vi "Official Gyro Example.vi"() -> ()   [LabVIEW 2016]
doc: "This example is for the HiTechnic Gyro Sensor together with the LEGO MINDSTORMS NXT. This program shows the angular rate on the NXT screen as well as on the Front Panel with a gauge indicator."
uses:
  <vilib>/NXT/HiTechnic/HiTechnic Controls/HiTechnic Port.ctl
  <vilib>/NXT/Block Support/NXT_InputPort.ctl
  <vilib>/NXT/Dual Mode Library/Display/drawText.vi
panel:
  out "Offset Value":i16
  in  "Reset Button":bool
  in  "stop":bool
  out "Gauge":i16(knob) scale=-360.0..360.0
  # "HiTechnic Gyro"
  # "Description\n\nThis example shows the HiTechnic Gyro Sensor value on the NXT screen on and this Front Panel gauge.  Pressing the Reset Offset button or the NXT Enter button will reset the Offset based on the current sensor reading.\n\nPorts\nPort 1: HiTechnic Gyro Sensor\n\n\nFor additional information: www.hitechnic.com"
  # "Controls and Indicators\n\nGauge shows the current Gyro Sensor value.  The units are in degrees/second.\n\nIf the sensor value is non-zero even when the sensor is not turning, press the Reset Offset button to adjust the offset."
  # "deg/sec"
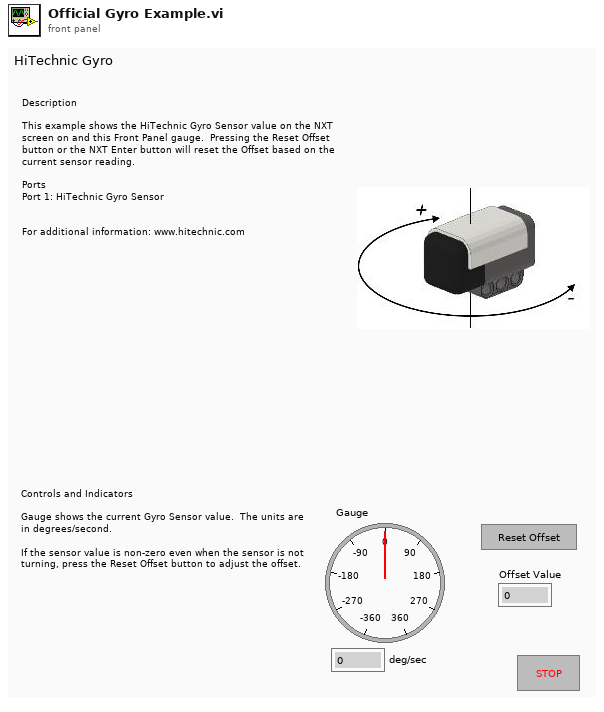
[diagram p1: front panel]
types:
  T1 = typedef "HiTechnic Port.ctl" = cluster{"Port":T2, "MUX Port":u8}
  T2 = typedef "NXT_InputPort.ctl" = u32
  T3 = typedef "LVHSConnector.ctl" = refnum<class "BrickReference.lvclass">
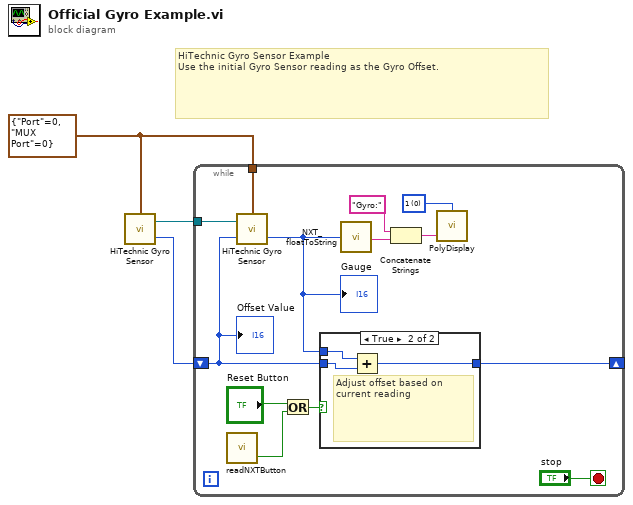
[diagram p0: block diagram]
diagram:
  w3 = T1 {"Port"=0, "MUX Port"=0} ("Port/MUX")
  # "HiTechnic Gyro Sensor Example\nUse the initial Gyro Sensor reading as the Gyro Offset."
  n1 = call <vilib>:"HiTechnic Gyro Sensor.vi"("Port/MUX"=w3) -> ("Gyro Value"=w1:i16, "NXT/EV3"=w2:T3)  [unwired: 2 in]
  n2 = while {
    tunnel: w3 -> [w11]
    tunnel: w2 -> [w10]
    shift-right: [w9] -> _
    shift-left: w1 -> [w8]
    stop <- "stop" stop-if-true
    w13 = i16 0 items=["1", "2", "3", "4", "5", "6", "7", "8"] ("Line")
    n3 = call <vilib>:"readNXTButton.vi"() -> ("Yes/No"=w4:bool)  [unwired: 3 in, 1 out]
    n4 = call <vilib>:"HiTechnic Gyro Sensor.vi"("Offset"=w8, "NXT/EV3"=w10, "Port/MUX"=w11) -> ("Gyro Value"=w7:i16)  [unwired: 1 out]
    "Gauge" <- w7
    n5 = Or(x="Reset Button", y=w4) -> (x .or. y?=w6:bool)
    n6 = case shown="True" w6 {
      tunnel: [w17 w20] -> w9
      tunnel: w8 -> [w17 w18]
      tunnel: w7 -> [_ w19]
      frame False {
      }
      frame True {
        # "Adjust offset based on current reading"
        n7 = Add(x=w19, y=w18) -> (x+y=w20:i16)
      }
    }
    n8 = call <vilib>:"NXT_floatToString.vi"("number"=w7) -> ("string"=w15:string)
    n9 = Concatenate Strings("Gyro:" ("string"), w15) -> (w14:string)
    n10 = call-poly <vilib>:"PolyDisplay.vi"("Text"=w14, "Line"=w13) -> ()  [unwired: 2 in, 1 out]
    "Offset Value" <- w8
  }
